vi "9213 16Ch TC Input.vi"(1 "9213 I/O":T1={"9213 TC0"="NI 9213/TC0", "9213 TC1"="NI 9213/TC1", "9213 TC2"="NI 9213/TC2", "9213 TC3"="NI 9213/TC3", "9213 TC4"="NI 9213/TC4", "9213 TC5"="NI 9213/TC5", "9213 TC6"="NI 9213/TC6", "9213 TC7"="NI 9213/TC7", "9213 TC8"="NI 9213/TC8", "9213 TC9"="NI 9213/TC9", "9213 TC10"="NI 9213/TC10", "9213 TC11"="NI 9213/TC11", "9213 TC12"="NI 9213/TC12", "9213 TC13"="NI 9213/TC13", "9213 TC14"="NI 9213/TC14", "9213 TC15"="NI 9213/TC15", "9213 CJC"="NI 9213/CJC", "9213 Autozero"="NI 9213/Autozero"}) -> (0 "Packets":u64[](array[numeric]))   [LabVIEW 2010]
uses:
  <vilib>/eio/EIONode/EIONode.xnode
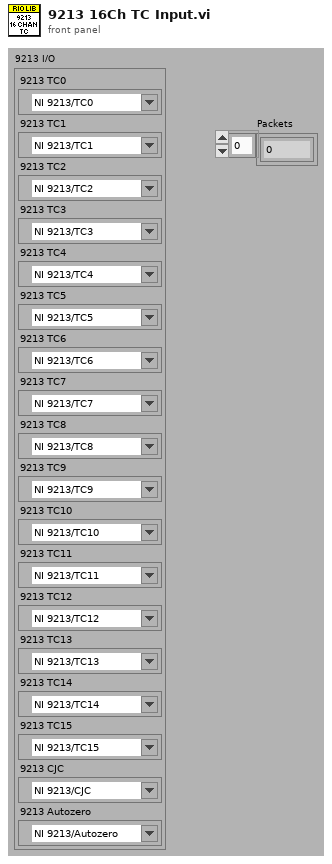
[diagram p1: front panel]
types:
  T1 = cluster{"9213 TC0":refnum<k21>, "9213 TC1":refnum<k21>, "9213 TC2":refnum<k21>, "9213 TC3":refnum<k21>, "9213 TC4":refnum<k21>, "9213 TC5":refnum<k21>, "9213 TC6":refnum<k21>, "9213 TC7":refnum<k21>, "9213 TC8":refnum<k21>, "9213 TC9":refnum<k21>, "9213 TC10":refnum<k21>, "9213 TC11":refnum<k21>, "9213 TC12":refnum<k21>, "9213 TC13":refnum<k21>, "9213 TC14":refnum<k21>, "9213 TC15":refnum<k21>, "9213 CJC":refnum<k21>, "9213 Autozero":refnum<k21>}
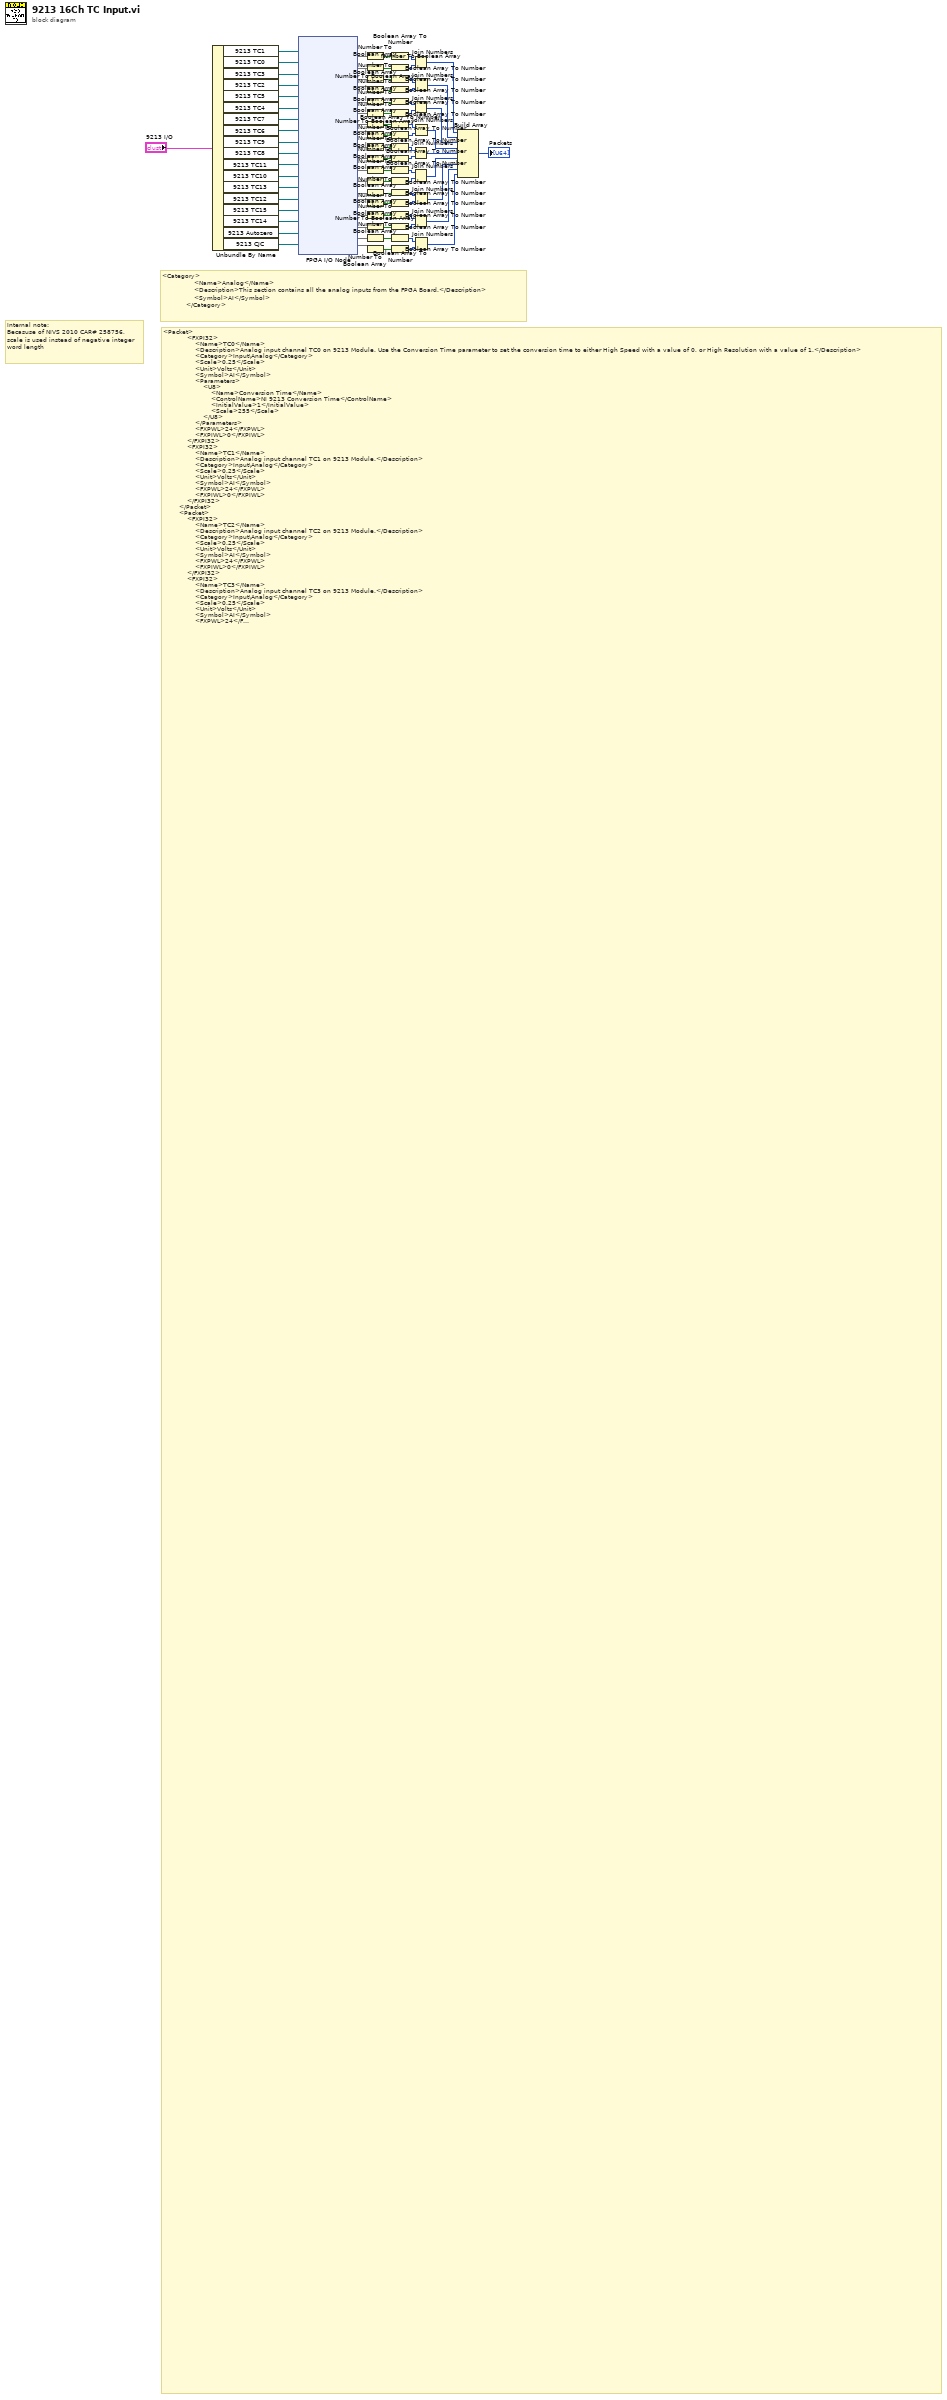
[diagram p0: block diagram]
diagram:
  # "Internal note:\nBecasuse of NIVS 2010 CAR# 258756, scale is used instead of negative integer word length"
  # "<Category>\n                <Name>Analog</Name>\n                <Description>This section contains all the analog inputs from the FPGA Board.</Description>\n                <Symbol>AI</Symbol>\n            </Category>"
  # "<Packet>\n            <FXPI32>\n                <Name>TC0</Name>\n                <Description>Analog input channel TC0 on 9213 Module. Use the Conversion Time parameter to set the conversion time to either High Speed with a value of 0, or High Resolution with a value of 1.</Description>\n                <Category>Input\\Analog</Category>\n                <Scale>0.25</Scale>\n                <Unit>Volts</Unit>\n                <Symbol>AI</Symbol>\n                <Parameters>\n                    <U8>\n                        <Name>Conversion Time</Name>\n                        <ControlName>NI 9213 Conversion Time</ControlName>\n                        <InitialValue>1</InitialValue>\n                        <Scale>255</Scale>\n                    </U8>\n                </Parameters>\n                <FXPWL>24</FXPWL>\n                <FXPIWL>0</FXPIWL>\n            </FXPI32>\n            <FXPI32>\n                <Name>TC1</Name>\n                <Description>Analog input channel TC1 on 9213 Module.</Description>\n                <Category>Input\\Analog</Category>\n                <Scale>0.25</Scale>\n                <Unit>Volts</Unit>\n                <Symbol>AI</Symbol>\n                <FXPWL>24</FXPWL>\n                <FXPIWL>0</FXPIWL>\n            </FXPI32>\n        </Packet>\n        <Packet>\n            <FXPI32>\n                <Name>TC2</Name>\n                <Description>Analog input channel TC2 on 9213 Module.</Description>\n                <Category>Input\\Analog</Category>\n                <Scale>0.25</Scale>\n                <Unit>Volts</Unit>\n                <Symbol>AI</Symbol>\n                <FXPWL>24</FXPWL>\n                <FXPIWL>0</FXPIWL>\n            </FXPI32>\n            <FXPI32>\n                <Name>TC3</Name>\n                <Description>Analog input channel TC3 on 9213 Module.</Description>\n                <Category>Input\\Analog</Category>\n                <Scale>0.25</Scale>\n                <Unit>Volts</Unit>\n                <Symbol>AI</Symbol>\n                <FXPWL>24</FXPWL>\n                <FXPIWL>0</FXPIWL>\n            </FXPI32>\n        </Packet>\n        <Packet>\n            <FXPI32>\n                <Name>TC4</Name>\n                <Description>Analog input channel TC4 on 9213 Module.</Description>\n                <Category>Input\\Analog</Category>\n                <Scale>0.25</Scale>\n                <Unit>Volts</Unit>\n                <Symbol>AI</Symbol>\n                <FXPWL>24</FXPWL>\n                <FXPIWL>0</FXPIWL>\n            </FXPI32>\n            <FXPI32>\n                <Name>TC5</Name>\n                <Description>Analog input channel TC5 on 9213 Module.</Description>\n                <Category>Input\\Analog</Category>\n                <Scale>0.25</Scale>\n                <Unit>Volts</Unit>\n                <Symbol>AI</Symbol>\n                <FXPWL>24</FXPWL>\n                <FXPIWL>0</FXPIWL>\n            </FXPI32>\n        </Packet>\n        <Packet>\n            <FXPI32>\n                <Name>TC6</Name>\n                <Description>Analog input channel TC6 on 9213 Module.</Description>\n                <Category>Input\\Analog</Category>\n                <Scale>0.25</Scale>\n                <Unit>Volts</Unit>\n                <Symbol>AI</Symbol>\n                <FXPWL>24</FXPWL>\n                <FXPIWL>0</FXPIWL>\n            </FXPI32>\n            <FXPI32>\n                <Name>TC7</Name>\n                <Description>Analog input channel TC7 on 9213 Module.</Description>\n                <Category>Input\\Analog</Category>\n                <Scale>0.25</Scale>\n                <Unit>Volts</Unit>\n                <Symbol>AI</Symbol>\n                <FXPWL>24</FXPWL>\n                <FXPIWL>0</FXPIWL>\n            </FXPI32>\n        </Packet>\n        <Packet>\n            <FXPI32>\n                <Name>TC8</Name>\n                <Description>Analog input channel TC8 on 9213 Module.</Description>\n                <Category>Input\\Analog</Category>\n                <Scale>0.25</Scale>\n                <Unit>Volts</Unit>\n                <Symbol>AI</Symbol>\n                <FXPWL>24</FXPWL>\n                <FXPIWL>0</FXPIWL>\n            </FXPI32>\n            <FXPI32>\n                <Name>TC9</Name>\n                <Description>Analog input channel TC9 on 9213 Module.</Description>\n                <Category>Input\\Analog</Category>\n                <Scale>0.25</Scale>\n                <Unit>Volts</Unit>\n                <Symbol>AI</Symbol>\n                <FXPWL>24</FXPWL>\n                <FXPIWL>0</FXPIWL>\n            </FXPI32>\n        </Packet>\n        <Packet>\n            <FXPI32>\n                <Name>TC10</Name>\n                <Description>Analog input channel TC10 on 9213 Module.</Description>\n                <Category>Input\\Analog</Category>\n                <Scale>0.25</Scale>\n                <Unit>Volts</Unit>\n                <Symbol>AI</Symbol>\n                <FXPWL>24</FXPWL>\n                <FXPIWL>0</FXPIWL>\n            </FXPI32>\n            <FXPI32>\n                <Name>TC11</Name>\n                <Description>Analog input channel TC11 on 9213 Module.</Description>\n                <Category>Input\\Analog</Category>\n                <Scale>0.25</Scale>\n                <Unit>Volts</Unit>\n                <Symbol>AI</Symbol>\n                <FXPWL>24</FXPWL>\n                <FXPIWL>0</FXPIWL>\n            </FXPI32>\n        </Packet>\n        <Packet>\n            <FXPI32>\n                <Name>TC12</Name>\n                <Description>Analog input channel TC12 on 9213 Module.</Description>\n                <Category>Input\\Analog</Category>\n                <Scale>0.25</Scale>\n                <Unit>Volts</Unit>\n                <Symbol>AI</Symbol>\n                <FXPWL>24</FXPWL>\n                <FXPIWL>0</FXPIWL>\n            </FXPI32>\n            <FXPI32>\n                <Name>TC13</Name>\n                <Description>Analog input channel TC13 on 9213 Module.</Description>\n                <Category>Input\\Analog</Category>\n                <Scale>0.25</Scale>\n                <Unit>Volts</Unit>\n                <Symbol>AI</Symbol>\n                <FXPWL>24</FXPWL>\n                <FXPIWL>0</FXPIWL>\n            </FXPI32>\n        </Packet>\n        <Packet>\n            <FXPI32>\n                <Name>TC14</Name>\n                <Description>Analog input channel TC14 on 9213 Module.</Description>\n                <Category>Input\\Analog</Category>\n                <Scale>0.25</Scale>\n                <Unit>Volts</Unit>\n                <Symbol>AI</Symbol>\n                <FXPWL>24</FXPWL>\n                <FXPIWL>0</FXPIWL>\n            </FXPI32>\n            <FXPI32>\n                <Name>TC15</Name>\n                <Description>Analog input channel TC15 on 9213 Module.</Description>\n                <Category>Input\\Analog</Category>\n                <Scale>0.25</Scale>\n                <Unit>Volts</Unit>\n                <Symbol>AI</Symbol>\n                <FXPWL>24</FXPWL>\n                <FXPIWL>0</FXPIWL>\n            </FXPI32>\n        </Packet>\n        <Packet>\n            <FXPI32>\n                <Name>CJC</Name>\n                <Description>Analog input channel CJC on 9213 Module.</Description>\n                <Category>Input\\Analog</Category>\n                <Scale>0.25</Scale>\n                <Unit>Volts</Unit>\n                <Symbol>AI</Symbol>\n                <FXPWL>24</FXPWL>\n                <FXPIWL>0</FXPIWL>\n            </FXPI32>\n            <FXPI32>\n                <Name>Autozero</Name>\n                <Description>Analog input channel Autozero on 9213 Module.</Description>\n                <Category>Input\\Analog</Category>\n                <Scale>0.25</Scale>\n                <Unit>Volts</Unit>\n                <Symbol>AI</Symbol>\n                <FXPWL>24</FXPWL>\n                <FXPIWL>0</FXPIWL>\n            </FXPI32>\n        </Packet>"
  n1 = Unbundle By Name("9213 I/O") -> ("9213 TC1"=w73:refnum<k21>, "9213 TC0"=w74:refnum<k21>, "9213 TC3"=w75:refnum<k21>, "9213 TC2"=w68:refnum<k21>, "9213 TC5"=w56:refnum<k21>, "9213 TC4"=w55:refnum<k21>, "9213 TC7"=w53:refnum<k21>, "9213 TC6"=w54:refnum<k21>, "9213 TC9"=w29:refnum<k21>, "9213 TC8"=w30:refnum<k21>, "9213 TC11"=w31:refnum<k21>, "9213 TC10"=w32:refnum<k21>, "9213 TC13"=w33:refnum<k21>, "9213 TC12"=w34:refnum<k21>, "9213 TC15"=w35:refnum<k21>, "9213 TC14"=w36:refnum<k21>, "9213 Autozero"=w37:refnum<k21>, "9213 CJC"=w38:refnum<k21>)
  n2 = xnode "FPGA I/O Node"("FPGA I/O In"=w73, "FPGA I/O In"=w74, "FPGA I/O In"=w75, "FPGA I/O In"=w68, "FPGA I/O In"=w56, "FPGA I/O In"=w55, "FPGA I/O In"=w53, "FPGA I/O In"=w54, "FPGA I/O In"=w29, "FPGA I/O In"=w30, "FPGA I/O In"=w31, "FPGA I/O In"=w32, "FPGA I/O In"=w33, "FPGA I/O In"=w34, "FPGA I/O In"=w35, "FPGA I/O In"=w36, "FPGA I/O In"=w37, "FPGA I/O In"=w38) -> ("I/O Item"=w79, "I/O Item"=w80, "I/O Item"=w65, "I/O Item"=w67, "I/O Item"=w59, "I/O Item"=w58, "I/O Item"=w44, "I/O Item"=w43, "I/O Item"=w42, "I/O Item"=w41, "I/O Item"=w12, "I/O Item"=w11, "I/O Item"=w10, "I/O Item"=w9, "I/O Item"=w8, "I/O Item"=w7, "I/O Item"=w6, "I/O Item"=w5)  [unwired: 18 out]
  n3 = Number To Boolean Array(number=w79) -> (Boolean array=w76:bool[])
  n4 = Number To Boolean Array(number=w80) -> (Boolean array=w77:bool[])
  n5 = Number To Boolean Array(number=w65) -> (Boolean array=w64:bool[])
  n6 = Number To Boolean Array(number=w67) -> (Boolean array=w78:bool[])
  n7 = Number To Boolean Array(number=w59) -> (Boolean array=w63:bool[])
  n8 = Number To Boolean Array(number=w58) -> (Boolean array=w62:bool[])
  n9 = Number To Boolean Array(number=w44) -> (Boolean array=w48:bool[])
  n10 = Number To Boolean Array(number=w43) -> (Boolean array=w46:bool[])
  n11 = Number To Boolean Array(number=w42) -> (Boolean array=w49:bool[])
  n12 = Number To Boolean Array(number=w41) -> (Boolean array=w50:bool[])
  n13 = Number To Boolean Array(number=w12) -> (Boolean array=w18:bool[])
  n14 = Number To Boolean Array(number=w11) -> (Boolean array=w17:bool[])
  n15 = Number To Boolean Array(number=w10) -> (Boolean array=w20:bool[])
  n16 = Number To Boolean Array(number=w9) -> (Boolean array=w16:bool[])
  n17 = Number To Boolean Array(number=w8) -> (Boolean array=w21:bool[])
  n18 = Number To Boolean Array(number=w7) -> (Boolean array=w22:bool[])
  n19 = Number To Boolean Array(number=w6) -> (Boolean array=w25:bool[])
  n20 = Number To Boolean Array(number=w5) -> (Boolean array=w27:bool[])
  n21 = Boolean Array To Number(Boolean array=w76) -> (number=w81:u32)
  n22 = Boolean Array To Number(Boolean array=w77) -> (number=w82:u32)
  n23 = Boolean Array To Number(Boolean array=w64) -> (number=w66:u32)
  n24 = Boolean Array To Number(Boolean array=w78) -> (number=w83:u32)
  n25 = Boolean Array To Number(Boolean array=w63) -> (number=w61:u32)
  n26 = Boolean Array To Number(Boolean array=w62) -> (number=w60:u32)
  n27 = Boolean Array To Number(Boolean array=w48) -> (number=w47:u32)
  n28 = Boolean Array To Number(Boolean array=w46) -> (number=w45:u32)
  n29 = Boolean Array To Number(Boolean array=w49) -> (number=w51:u32)
  n30 = Boolean Array To Number(Boolean array=w50) -> (number=w52:u32)
  n31 = Boolean Array To Number(Boolean array=w18) -> (number=w15:u32)
  n32 = Boolean Array To Number(Boolean array=w17) -> (number=w14:u32)
  n33 = Boolean Array To Number(Boolean array=w20) -> (number=w19:u32)
  n34 = Boolean Array To Number(Boolean array=w16) -> (number=w13:u32)
  n35 = Boolean Array To Number(Boolean array=w21) -> (number=w23:u32)
  n36 = Boolean Array To Number(Boolean array=w22) -> (number=w24:u32)
  n37 = Boolean Array To Number(Boolean array=w25) -> (number=w26:u32)
  n38 = Boolean Array To Number(Boolean array=w27) -> (number=w28:u32)
  n39 = Join Numbers(hi=w81, lo=w82) -> ((hi.lo)=w71:u64)
  n40 = Join Numbers(hi=w61, lo=w60) -> ((hi.lo)=w57:u64)
  n41 = Join Numbers(hi=w51, lo=w52) -> ((hi.lo)=w40:u64)
  n42 = Join Numbers(hi=w15, lo=w14) -> ((hi.lo)=w1:u64)
  n43 = Join Numbers(hi=w23, lo=w24) -> ((hi.lo)=w3:u64)
  n44 = Join Numbers(hi=w66, lo=w83) -> ((hi.lo)=w72:u64)
  n45 = Join Numbers(hi=w47, lo=w45) -> ((hi.lo)=w39:u64)
  n46 = Join Numbers(hi=w19, lo=w13) -> ((hi.lo)=w2:u64)
  n47 = Join Numbers(hi=w26, lo=w28) -> ((hi.lo)=w4:u64)
  n48 = Build Array(w71, w72, w57, w39, w40, w1, w2, w3, w4) -> (→"Packets":u64[])
